vi "Publisher Do.vi"(8 "error in (no error)":errorcluster, 10 "Publisher in":refnum<class "Publisher.lvclass">, 11 "Subscribe Msg":refnum<class "Sender Msg.lvclass">) -> (0 "error out":errorcluster, 2 "Publisher out":refnum<class "Publisher.lvclass">)   [LabVIEW 2020, in "Publisher.lvlib" / "Sender Msg.lvclass"]
doc: "This VI delivers the message to the actor by calling the appropriate method(s) on the actor.\n\nThis implementation drops messages by default."
uses:
  Sender Msg.lvclass
  Publisher/Publisher.lvclass
  Sender Msg.lvclass/Sender Msg.ctl
  PPL/HDH.Actor Framework.Core.Actor.lvlibp/1abvi3w/vi.lib/ActorFramework/Message/Message.lvclass
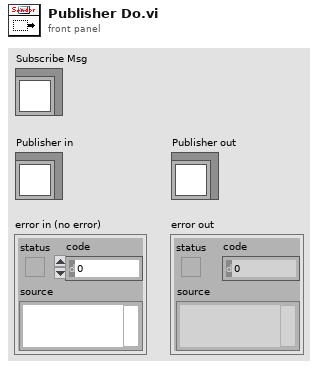
[diagram p1: front panel]
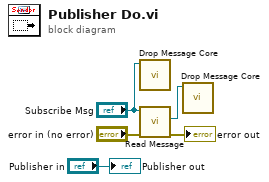
[diagram p0: block diagram]
diagram:
  n1 = call-dynamic "Drop Message Core.vi"("Message in"="Subscribe Msg") -> ()  [unwired: 11 in]
  n2 = call "Read Message.vi"("error in (no error)"="error in (no error)", "Sender Msg in"="Subscribe Msg") -> ("error out"=→"error out":errorcluster, "Message"=w3:refnum<class "Message.lvclass">)  [unwired: 7 in, 1 out]
  n3 = call-dynamic "Drop Message Core.vi"("Message in"=w3) -> ()  [unwired: 11 in]
  "Publisher out" <- "Publisher in"
